vi "read_params.vi"(8 "error in (no error)":errorcluster, 11 "MiniBatchKMeans in":refnum<class "MiniBatchKMeans.lvclass">) -> (0 "error out":errorcluster, 2 "params":T1={"n_clusters"=8.0, "init"={"init_type"="k-means++", "init_list"=[]}, "max_iter"=100.0, "batch_size"=100.0, "verbose"=0.0, "compute_labels"=TRUE, "random_state"=0.0, "tol"=0.0, "max_no_improvement"=10.0, "init_size"={"init_size_type"="None", "init_size_int"=0.0}, "n_init"=3.0, "reassignment_ratio"=0.01}, 3 "MiniBatchKMeans out":refnum<class "MiniBatchKMeans.lvclass">)   [LabVIEW 2020, in "MiniBatchKMeans.lvclass"]
uses:
  MiniBatchKMeans.lvclass
  Controls/mini_batch_kmeans_params.ctl
  MiniBatchKMeans.lvclass/MiniBatchKMeans.ctl
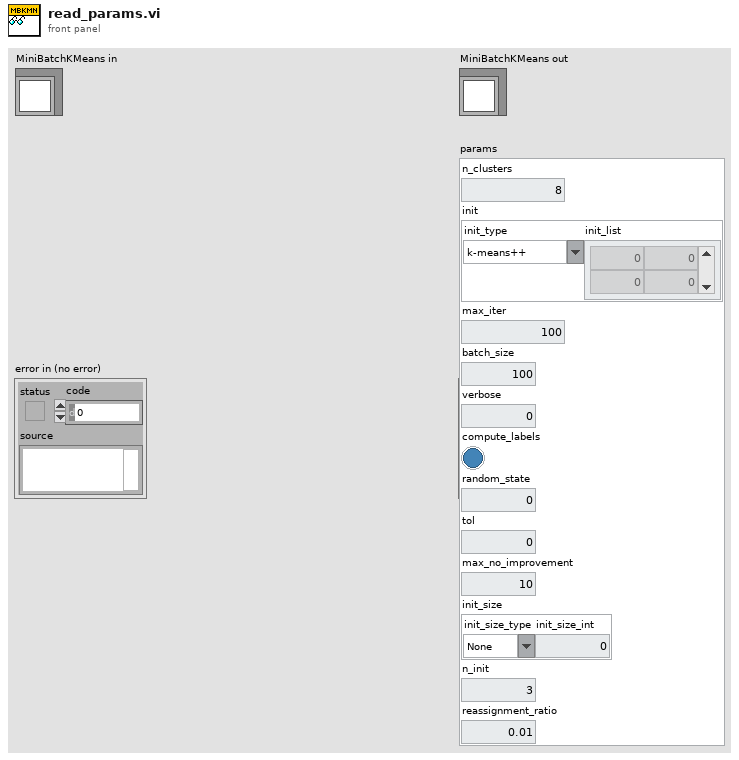
[diagram p1: front panel]
types:
  T1 = typedef "mini_batch_kmeans_params.ctl" = cluster{"n_clusters":dbl, "init":cluster{"init_type":string, "init_list":dbl[][]}, "max_iter":dbl, "batch_size":dbl, "verbose":dbl, "compute_labels":bool, "random_state":dbl, "tol":dbl, "max_no_improvement":dbl, "init_size":cluster{"init_size_type":string, "init_size_int":dbl}, "n_init":dbl, "reassignment_ratio":dbl}
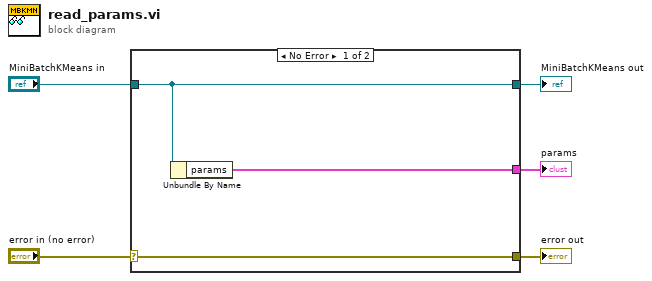
[diagram p0: block diagram]
diagram:
  n1 = case shown="No Error" "error in (no error)" {
    selector: "error in (no error)" -> [w8 w9]
    tunnel: [w8 w9] -> w4
    tunnel: [w7 w10] -> w2
    tunnel: "MiniBatchKMeans in" -> [w7 w10]
    tunnel: [w6 _] -> w1
    frame No Error {
      n2 = Unbundle By Name(w7) -> ("params"=w6:T1)
    }
    frame Error {
    }
  }
  "error out" <- w4
  "MiniBatchKMeans out" <- w2
  "params" <- w1
